vi "I2C_Core_[Top-Level].vi"() -> ()   [LabVIEW 2019]
doc: "I2C Core is a general FPGA VI for communicating with I2C devices.\n_____________________________________________________\nI2C Data transfers fit into three basic formats: \n\nThe first, a simple master-to-slave transfer, begins with the master generating a start condition. The master then sends the desired 7-bit slave address with the read/write bit cleared and begins the acknowledgment clock cycle. Once the ACK condition is observed, the cycle of writing data and reading ACK bits continues until the receiver either issues a NOACK or the transmitter completes the transfer and issues a STOP condition. \n\nThe second format, master-slave read, is similar to the previous format, except that the slave device immediately begins placing data onto the bus after the acknowledgment clock. \n\nThe last category is a combined format. Often this format is used when a device requires some initial configuration information in order to continue. Again, this format is similar to the previous two except that instead of issuing a stop condition, the transmitter issues a second start condition, followed by the slave address. You will often see this command used when accessing devices like serial EEPROMs. The first sequence is used to supply the device with the address that should be read, while the second start and clock sequence are used to clock the data back. \n\n\nTechnical Information Source:\nhttp://www.embedded.com/97/feat9711.htm\n_____________________________________________________\n\nWritten By: \nPeter Fuller\nplf Consulting, LLC\n258 Harvard St #324\nBrookline, MA 02446\n\nemail: peter@plfconsulting.com\nphone: 617.699.2201"
uses:
  Controls/i2c_state.ctl
  <vilib>/eio/EIONode/EIONode.xnode
  Instance           4 28Saved   I2C_Core_[Top-Level] .vi
  <vilib>/eio/EIOMethodNode/EIOMethodNode.xnode
  <vilib>/rvi/eio/common/nirviEmuTemplateMethod_errors.vi
panel:
  out "AI3":fxp<+/-,24,5>
  out "AI2":fxp<+/-,24,5>
  out "AI1":fxp<+/-,24,5>
  in  "Execute 2":bool
  in  "HalfCycle(Ticks) 2":u32=200
  in  "i2c_State 2":T1=enum."W_To_Device"
  in  "Address 2":u8 format="%08x"
  in  "10-bitAddress 2":u8 format="%08b"
  in  "TransmitDelay(Ticks) 2":u32=1000
  in  "Use_10-Bit_Address 2":bool
  in  "StartStopDelay(Ticks) 2":u32=1200
  in  "PostAddressDelay(Ticks) 2":u32=1200
  in  "NumBytesToWrite 2":i32
  in  "NumBytesToRead 2":i32
  out "error 2":errorcluster
  out "Status 2":i16
  in  "CMD/Param 2":u8 format="%.0x"
  out "Data 2":u8 format="%.0x"
  in  "MemoryAddress 2":u32
  in  "GetRead 2":bool
  in  "UpdateWrite 2":bool
  out "AI0":fxp<+/-,24,5>
  out "error":errorcluster
  in  "PostAddressDelay(Ticks)":u32=1200
  in  "StartStopDelay(Ticks)":u32=1200
  in  "NumBytesToRead":i32
  in  "NumBytesToWrite":i32
  in  "UpdateWrite":bool
  in  "GetRead":bool
  in  "CMD/Param":u8 format="%.0x"
  out "Data":u8 format="%.0x"
  in  "MemoryAddress":u32
  out "Status":i16
  in  "Use_10-Bit_Address":bool
  in  "TransmitDelay(Ticks)":u32=1000
  in  "10-bitAddress":u8 format="%08b"
  in  "Address":u8 format="%08x"
  in  "HalfCycle(Ticks)":u32=200
  in  "i2c_State":T1=enum."W_To_Device"
  in  "Execute":bool
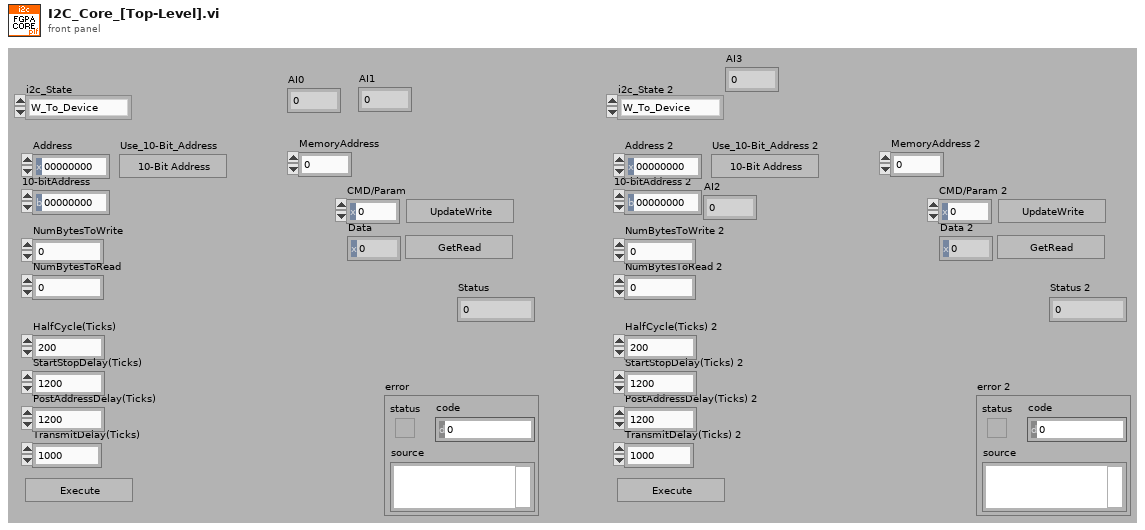
[diagram p1: front panel]
types:
  T1 = typedef "i2c_state.ctl" = enum16{"Monitor", "W_To_Device", "R_From_Device", "W/R_From_Device", "TerminateCore"}
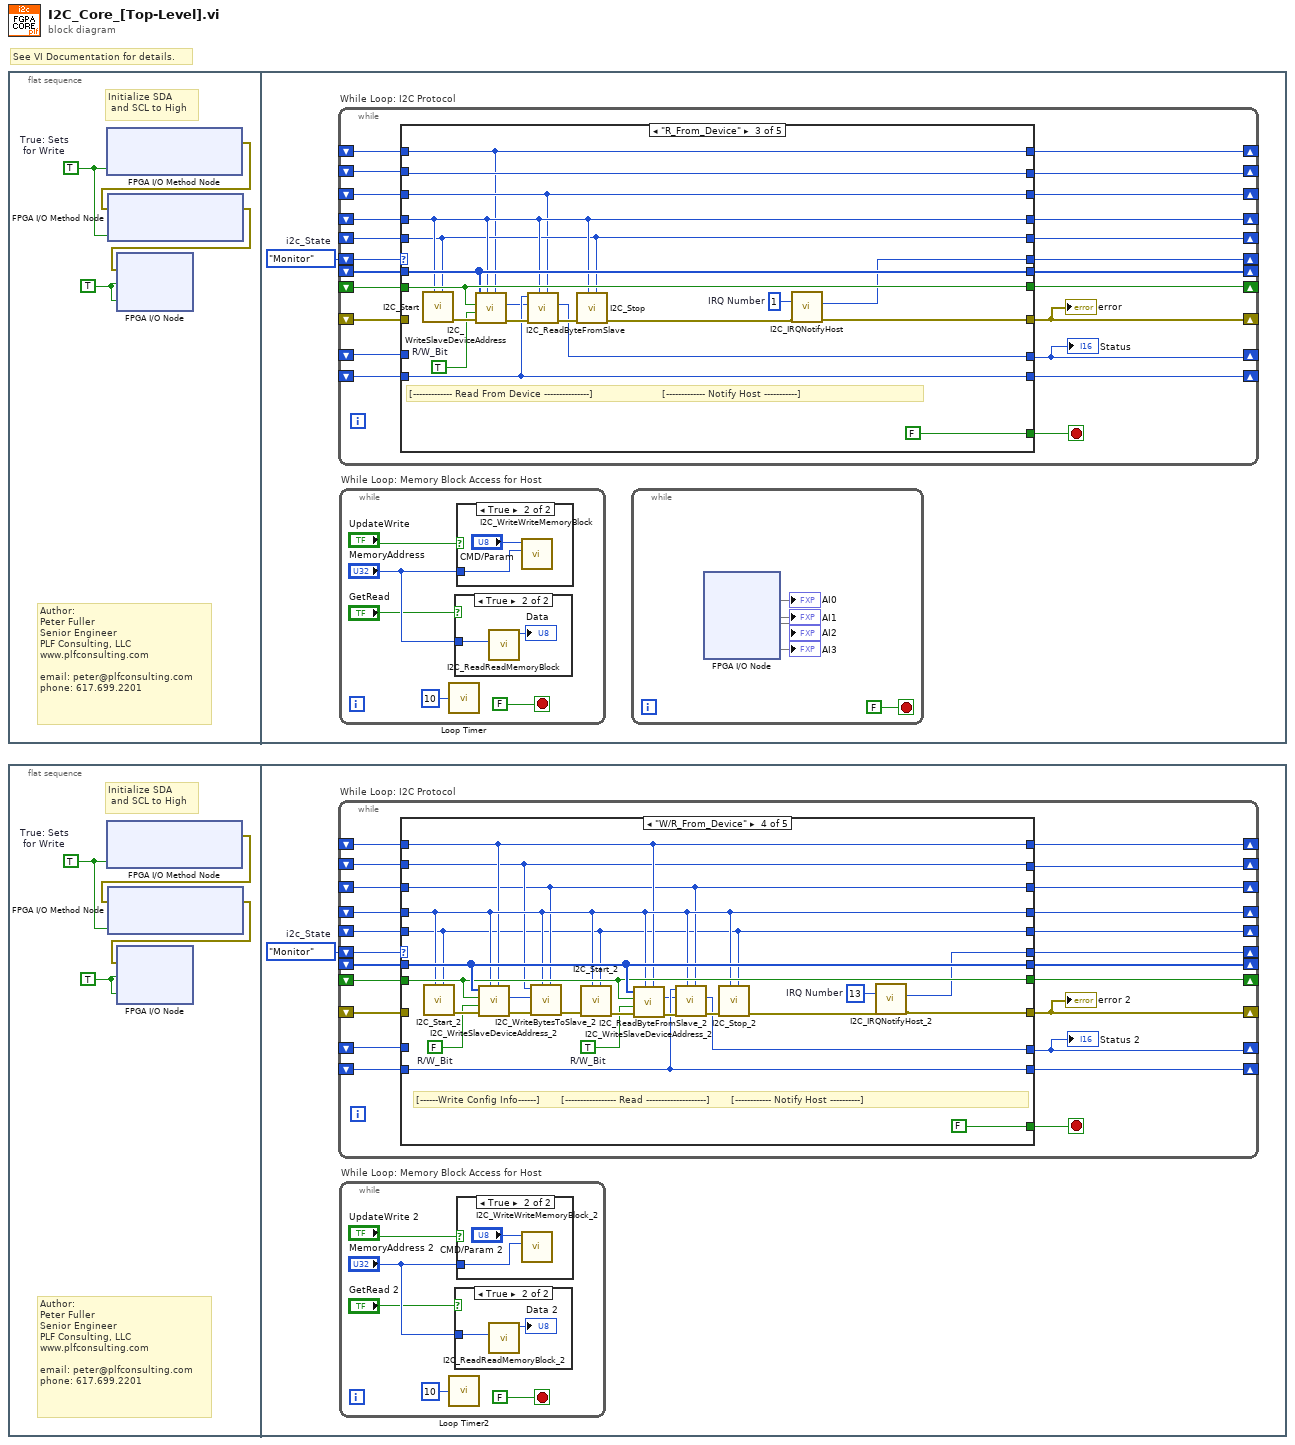
[diagram p0: block diagram]
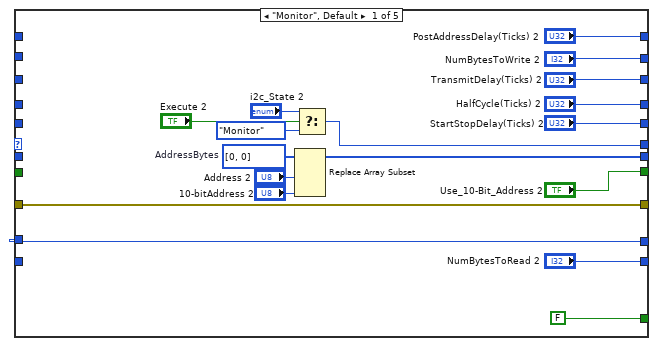
[diagram p4: hidden frame]
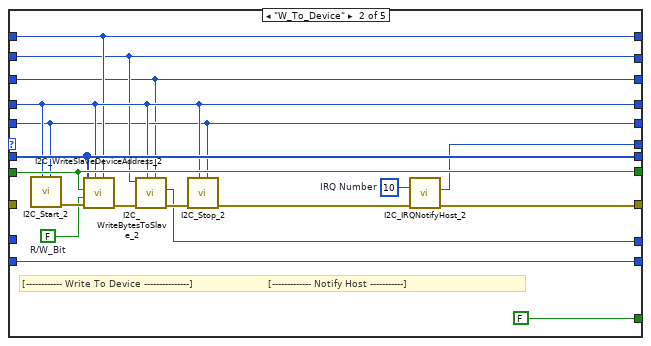
[diagram p5: hidden frame]
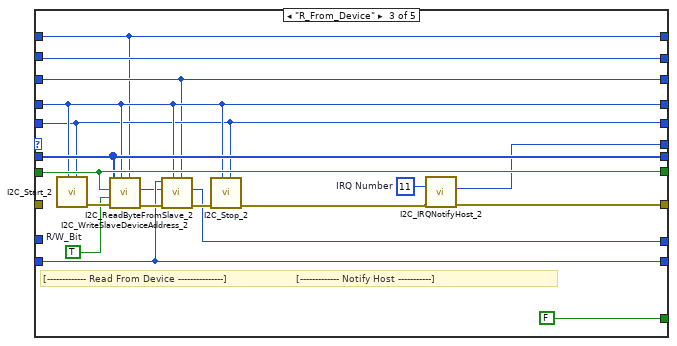
[diagram p6: hidden frame]
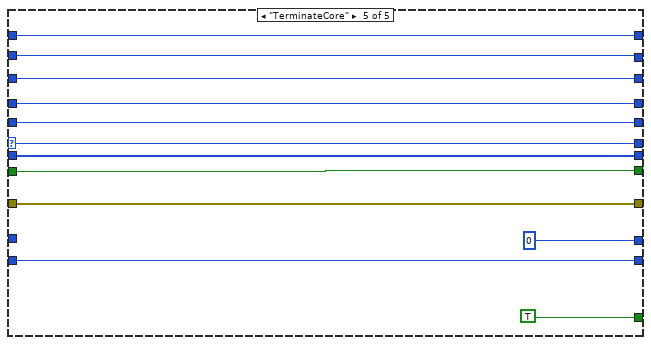
[diagram p7: hidden frame]
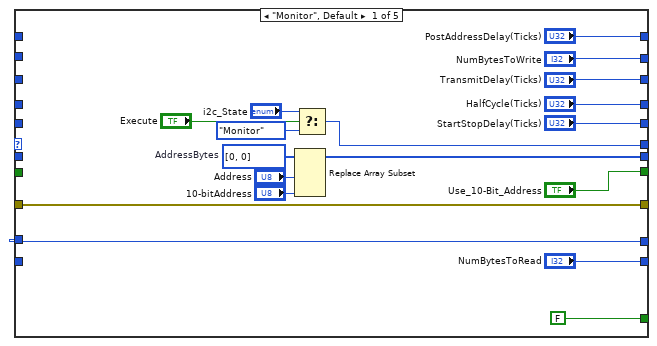
[diagram p10: hidden frame]
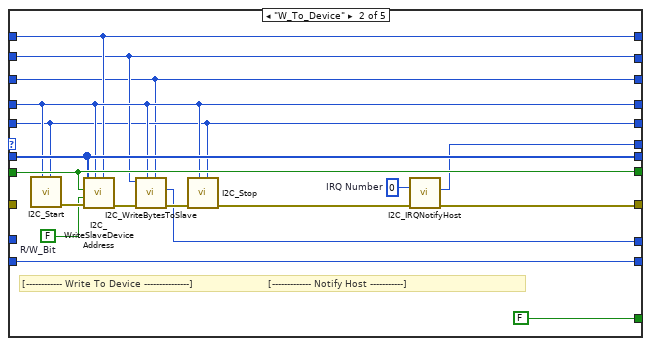
[diagram p11: hidden frame]
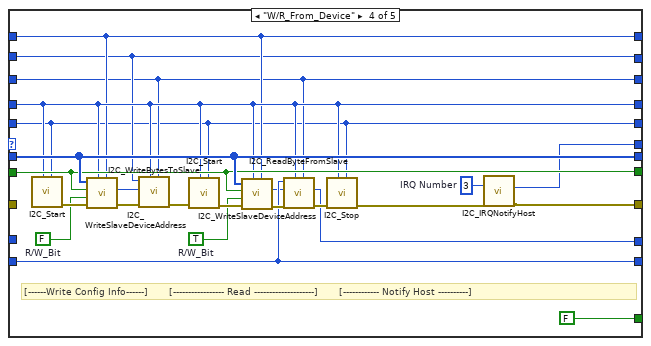
[diagram p12: hidden frame]
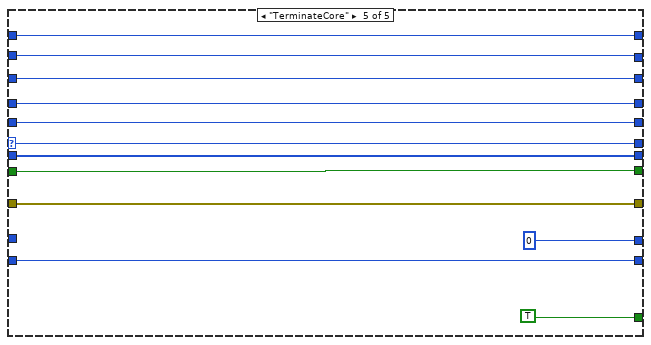
[diagram p13: hidden frame]
diagram:
  # "See VI Documentation for details."
  n1 = flat-sequence {
    frame #0 {
      w2 = TRUE  # True: Sets   for Write
      w4 = TRUE ("SDA")
      # "Author:\nPeter Fuller\nSenior Engineer\nPLF Consulting, LLC\nwww.plfconsulting.com\n\nemail: peter@plfconsulting.com\nphone: 617.699.2201"
      # "Initialize SDA\n and SCL to High"
      n2 = xnode "FPGA I/O Method Node"("Enable"=w2) -> ("error out"=w3:errorcluster)  [unwired: 2 in, 1 out]
      n3 = xnode "FPGA I/O Method Node"("error in"=w3, "Enable"=w2) -> ("error out"=w1:errorcluster)  [unwired: 1 in, 1 out]
      n4 = xnode "FPGA I/O Node"("error in"=w1, "SDA"=w4, "SCL"=w4) -> ()  [unwired: 2 in, 3 out]
    }
    frame #1 {
      w5 = i2c_state."Monitor"  # i2c_State
      n5 = while "While Loop: I2C Protocol" {
        shift-right: [w37] -> _
        shift-left: w5 -> [w38]
        shift-right: [w41] -> _
        shift-left: _ -> [w42]
        shift-right: [w22] -> _
        shift-left: _ -> [w40]
        shift-right: [w36] -> _
        shift-left: _ -> [w39]
        shift-right: [w35] -> _
        shift-left: _ -> [w34]
        shift-right: [w33] -> _
        shift-left: _ -> [w32]
        shift-right: [w30] -> _
        shift-left: _ -> [w26]
        shift-right: [w29] -> _
        shift-left: _ -> [w25]
        shift-right: [w28] -> _
        shift-left: _ -> [w23]
        shift-right: [w27] -> _
        shift-left: _ -> [w24]
        shift-right: [w21] -> _
        shift-left: _ -> [w20]
        stop <- w31 stop-if-true
        n6 = case shown="\"R_From_Device\"" w38 {
          selector: w38 -> [_ _ _ _ w126]
          tunnel: ["HalfCycle(Ticks)" w75 w92 w113 w128] -> w41
          tunnel: w42 -> [_ w75 w92 w113 w128]
          tunnel: [w56 w70 w79 w98 w126] -> w37
          tunnel: w40 -> [w44 _ _ _ w132]
          tunnel: [w44 w63 w80 w99 w132] -> w22
          tunnel: w39 -> [_ w76 w95 w118 w125]
          tunnel: [w52 w76 w95 w118 w125] -> w36
          tunnel: ["Use_10-Bit_Address" w77 w96 w117 w124] -> w35
          tunnel: w34 -> [_ w77 w96 w117 w124]
          tunnel: ["TransmitDelay(Ticks)" w64 w86 w106 w129] -> w33
          tunnel: w32 -> [_ w64 w86 w106 w129]
          tunnel: [FALSE FALSE FALSE FALSE TRUE] -> w31
          tunnel: w25 -> [_ w67 w89 w108 w130]
          tunnel: w24 -> [_ w66 w88 w107 w123]
          tunnel: w23 -> [_ w65 w87 w105 w127]
          tunnel: ["PostAddressDelay(Ticks)" w68 w85 w109 w131] -> w30
          tunnel: ["NumBytesToWrite" w67 w89 w108 w130] -> w29
          tunnel: ["StartStopDelay(Ticks)" w65 w87 w105 w127] -> w28
          tunnel: ["NumBytesToRead" w66 w88 w107 w123] -> w27
          tunnel: w26 -> [_ w68 w85 w109 w131]
          tunnel: [w43 w62 w84 w104 i16 0 ("Status")] -> w21
          tunnel: w20 -> [w43 _ _ _ _]
          frame "Monitor", Default {
            w55 = u8[] [0, 0]  # AddressBytes
            n7 = Replace Array Subset(array=w55, new element #1="Address", new element #2="10-bitAddress") -> (w52:u8[])  [unwired: 2 in]
            n8 = Select(t="i2c_State", s="Execute", f=i2c_state."Monitor") -> (s? t:f=w56:T1)
          }
          frame "W_To_Device" {
            w61 = u8 0  # IRQ Number
            w71 = FALSE  # R/W_Bit
            # "[------------ Write To Device ---------------]                         [------------- Notify Host -----------]"
            n9 = call "I2C_Start.vi"("TransmitDelay(Ticks)"=w65, "HalfCycle(Ticks)"=w75) -> ("error out"=w74:errorcluster)  [unwired: 2 in, 7 out]
            n10 = call "I2C_WriteSlaveDeviceAddress.vi"("PostAddressDelay(Ticks)"=w68, "HalfCycle(Ticks)"=w75, "error in"=w74, "R/W_Bit"=w71, "10-Bit Address"=w77, "AddressBits"=w76) -> ("error out"=w78:errorcluster)  [unwired: 5 out]
            n11 = call "I2C_WriteBytesToSlave.vi"("InterByteTransmitDelay(Ticks)"=w64, "HalfCycle(Ticks)"=w75, "error in"=w78, "NumBytesToWrite"=w67) -> ("error out"=w73:errorcluster, "Status"=w62:i16)  [unwired: 1 in, 5 out]
            n12 = call "I2C_Stop.vi"("TransmitDelay(Ticks)"=w65, "HalfCycle(Ticks)"=w75, "error in"=w73) -> ("error out"=w69:errorcluster)  [unwired: 1 in, 7 out]
            n13 = call "I2C_IRQNotifyHost.vi"("error out in"=w69, "IRQ Number"=w61) -> ("error out"=w63:errorcluster, "i2c_State"=w70:T1)  [unwired: 8 out]
          }
          frame "R_From_Device" {
            w82 = u8 1  # IRQ Number
            w90 = TRUE  # R/W_Bit
            # "[------------- Read From Device ---------------]                       [------------- Notify Host -----------]"
            n14 = call "I2C_Start.vi"("TransmitDelay(Ticks)"=w87, "HalfCycle(Ticks)"=w92) -> ("error out"=w94:errorcluster)  [unwired: 2 in, 7 out]
            n15 = call "I2C_WriteSlaveDeviceAddress.vi"("PostAddressDelay(Ticks)"=w85, "HalfCycle(Ticks)"=w92, "error in"=w94, "R/W_Bit"=w90, "10-Bit Address"=w96, "AddressBits"=w95) -> ("error out"=w97:errorcluster, "Status"=w83:i16)  [unwired: 4 out]
            n16 = call "I2C_ReadByteFromSlave.vi"("InterByteTransmitDelay(Ticks)"=w86, "HalfCycle(Ticks)"=w92, "error in"=w97, "StatusIn"=w83, "NumBytesToRead"=w88) -> ("error out"=w93:errorcluster, "Status"=w84:i16)  [unwired: 5 out]
            n17 = call "I2C_Stop.vi"("TransmitDelay(Ticks)"=w87, "HalfCycle(Ticks)"=w92, "error in"=w93) -> ("error out"=w81:errorcluster)  [unwired: 1 in, 7 out]
            n18 = call "I2C_IRQNotifyHost.vi"("error out in"=w81, "IRQ Number"=w82) -> ("error out"=w80:errorcluster, "i2c_State"=w79:T1)  [unwired: 8 out]
          }
          frame "W/R_From_Device" {
            w101 = u8 3  # IRQ Number
            w110 = TRUE  # R/W_Bit
            w111 = FALSE  # R/W_Bit
            # "[------Write Config Info------]       [----------------- Read --------------------]       [------------ Notify Host ----------]"
            n19 = call "I2C_Start.vi"("TransmitDelay(Ticks)"=w105, "HalfCycle(Ticks)"=w113) -> ("error out"=w121:errorcluster)  [unwired: 2 in, 7 out]
            n20 = call "I2C_WriteSlaveDeviceAddress.vi"("PostAddressDelay(Ticks)"=w109, "HalfCycle(Ticks)"=w113, "error in"=w121, "R/W_Bit"=w111, "10-Bit Address"=w117, "AddressBits"=w118) -> ("error out"=w114:errorcluster, "Status"=w103:i16)  [unwired: 4 out]
            n21 = call "I2C_WriteBytesToSlave.vi"("InterByteTransmitDelay(Ticks)"=w106, "HalfCycle(Ticks)"=w113, "error in"=w114, "StatusIn"=w103, "NumBytesToWrite"=w108) -> ("error out"=w115:errorcluster)  [unwired: 6 out]
            n22 = call "I2C_Start.vi"("TransmitDelay(Ticks)"=w105, "HalfCycle(Ticks)"=w113, "error in"=w115) -> ("error out"=w119:errorcluster)  [unwired: 1 in, 7 out]
            n23 = call "I2C_WriteSlaveDeviceAddress.vi"("PostAddressDelay(Ticks)"=w109, "HalfCycle(Ticks)"=w113, "error in"=w119, "R/W_Bit"=w110, "10-Bit Address"=w117, "AddressBits"=w118) -> ("error out"=w116:errorcluster, "Status"=w102:i16)  [unwired: 4 out]
            n24 = call "I2C_ReadByteFromSlave.vi"("InterByteTransmitDelay(Ticks)"=w106, "HalfCycle(Ticks)"=w113, "error in"=w116, "StatusIn"=w102, "NumBytesToRead"=w107) -> ("error out"=w120:errorcluster, "Status"=w104:i16)  [unwired: 5 out]
            n25 = call "I2C_Stop.vi"("TransmitDelay(Ticks)"=w105, "HalfCycle(Ticks)"=w113, "error in"=w120) -> ("error out"=w100:errorcluster)  [unwired: 1 in, 7 out]
            n26 = call "I2C_IRQNotifyHost.vi"("error out in"=w100, "IRQ Number"=w101) -> ("error out"=w99:errorcluster, "i2c_State"=w98:T1)  [unwired: 8 out]
          }
          frame "TerminateCore" {
          }
        }
        "error" <- w22
        "Status" <- w21
      }
      n27 = while "While Loop: Memory Block Access for Host" {
        stop <- FALSE stop-if-true
        n28 = call "Loop Timer"("Count(Ticks)"=u16 10) -> ()  [unwired: 1 out]
        n29 = case shown="True" "GetRead" {
          tunnel: "MemoryAddress" -> [_ w17]
          frame False {
          }
          frame True {
            n30 = call "I2C_ReadReadMemoryBlock.vi"("MemoryAddress"=w17) -> ("Data"=→"Data":u8)  [unwired: 1 in, 9 out]
          }
        }
        n31 = case shown="True" "UpdateWrite" {
          tunnel: "MemoryAddress" -> [_ w19]
          frame False {
          }
          frame True {
            n32 = call "I2C_WriteWriteMemoryBlock.vi"("MemoryAddress"=w19, "Data"="CMD/Param") -> ()  [unwired: 1 in, 9 out]
          }
        }
      }
      n33 = while {
        stop <- FALSE stop-if-true
        n34 = xnode "FPGA I/O Node"() -> ("AI0"=→"AI0", "AI1"=→"AI1", "AI2"=→"AI2", "AI3"=→"AI3")  [unwired: 4 in, 4 out]
      }
    }
  }
  n35 = flat-sequence {
    frame #0 {
      w135 = TRUE  # True: Sets   for Write
      w137 = TRUE ("SDA")
      # "Author:\nPeter Fuller\nSenior Engineer\nPLF Consulting, LLC\nwww.plfconsulting.com\n\nemail: peter@plfconsulting.com\nphone: 617.699.2201"
      # "Initialize SDA\n and SCL to High"
      n36 = xnode "FPGA I/O Method Node"("Enable"=w135) -> ("error out"=w136:errorcluster)  [unwired: 2 in, 1 out]
      n37 = xnode "FPGA I/O Method Node"("error in"=w136, "Enable"=w135) -> ("error out"=w134:errorcluster)  [unwired: 1 in, 1 out]
      n38 = xnode "FPGA I/O Node"("error in"=w134, "SDA2"=w137, "SCL2"=w137) -> ()  [unwired: 2 in, 3 out]
    }
    frame #1 {
      w138 = i2c_state."Monitor"  # i2c_State
      n39 = while "While Loop: I2C Protocol" {
        shift-right: [w165] -> _
        shift-left: w138 -> [w166]
        shift-right: [w169] -> _
        shift-left: _ -> [w170]
        shift-right: [w150] -> _
        shift-left: _ -> [w168]
        shift-right: [w164] -> _
        shift-left: _ -> [w167]
        shift-right: [w163] -> _
        shift-left: _ -> [w162]
        shift-right: [w161] -> _
        shift-left: _ -> [w160]
        shift-right: [w158] -> _
        shift-left: _ -> [w154]
        shift-right: [w157] -> _
        shift-left: _ -> [w153]
        shift-right: [w156] -> _
        shift-left: _ -> [w151]
        shift-right: [w155] -> _
        shift-left: _ -> [w152]
        shift-right: [w149] -> _
        shift-left: _ -> [w148]
        stop <- w159 stop-if-true
        n40 = case shown="\"W/R_From_Device\"" w166 {
          selector: w166 -> [_ _ _ _ w254]
          tunnel: ["HalfCycle(Ticks) 2" w203 w220 w241 w256] -> w169
          tunnel: w170 -> [_ w203 w220 w241 w256]
          tunnel: [w184 w198 w207 w226 w254] -> w165
          tunnel: w168 -> [w172 _ _ _ w260]
          tunnel: [w172 w191 w208 w227 w260] -> w150
          tunnel: w167 -> [_ w204 w223 w246 w253]
          tunnel: [w180 w204 w223 w246 w253] -> w164
          tunnel: ["Use_10-Bit_Address 2" w205 w224 w245 w252] -> w163
          tunnel: w162 -> [_ w205 w224 w245 w252]
          tunnel: ["TransmitDelay(Ticks) 2" w192 w214 w234 w257] -> w161
          tunnel: w160 -> [_ w192 w214 w234 w257]
          tunnel: [FALSE FALSE FALSE FALSE TRUE] -> w159
          tunnel: w153 -> [_ w195 w217 w236 w258]
          tunnel: w152 -> [_ w194 w216 w235 w251]
          tunnel: w151 -> [_ w193 w215 w233 w255]
          tunnel: ["PostAddressDelay(Ticks) 2" w196 w213 w237 w259] -> w158
          tunnel: ["NumBytesToWrite 2" w195 w217 w236 w258] -> w157
          tunnel: ["StartStopDelay(Ticks) 2" w193 w215 w233 w255] -> w156
          tunnel: ["NumBytesToRead 2" w194 w216 w235 w251] -> w155
          tunnel: w154 -> [_ w196 w213 w237 w259]
          tunnel: [w171 w190 w212 w232 i16 0 ("Status")] -> w149
          tunnel: w148 -> [w171 _ _ _ _]
          frame "Monitor", Default {
            w183 = u8[] [0, 0]  # AddressBytes
            n41 = Replace Array Subset(array=w183, new element #1="Address 2", new element #2="10-bitAddress 2") -> (w180:u8[])  [unwired: 2 in]
            n42 = Select(t="i2c_State 2", s="Execute 2", f=i2c_state."Monitor") -> (s? t:f=w184:T1)
          }
          frame "W_To_Device" {
            w189 = u8 10  # IRQ Number
            w199 = FALSE  # R/W_Bit
            # "[------------ Write To Device ---------------]                         [------------- Notify Host -----------]"
            n43 = call "I2C_Start_2.vi"("TransmitDelay(Ticks)"=w193, "HalfCycle(Ticks)"=w203) -> ("error out"=w202:errorcluster)  [unwired: 9 in]
            n44 = call "I2C_WriteSlaveDeviceAddress_2.vi"("PostAddressDelay(Ticks)"=w196, "HalfCycle(Ticks)"=w203, "error in"=w202, "R/W_Bit"=w199, "10-Bit Address"=w205, "AddressBits"=w204) -> ("error out"=w206:errorcluster)  [unwired: 4 in, 1 out]
            n45 = call "I2C_WriteBytesToSlave_2.vi"("InterByteTransmitDelay(Ticks)"=w192, "HalfCycle(Ticks)"=w203, "error in"=w206, "NumBytesToWrite"=w195) -> ("error out"=w201:errorcluster, "Status"=w190:i16)  [unwired: 6 in]
            n46 = call "I2C_Stop_2.vi"("TransmitDelay(Ticks)"=w193, "HalfCycle(Ticks)"=w203, "error in"=w201) -> ("error out"=w197:errorcluster)  [unwired: 8 in]
            n47 = call "I2C_IRQNotifyHost_2.vi"("error out in"=w197, "IRQ Number"=w189) -> ("error out"=w191:errorcluster, "i2c_State"=w198:T1)  [unwired: 8 in]
          }
          frame "R_From_Device" {
            w210 = u8 11  # IRQ Number
            w218 = TRUE  # R/W_Bit
            # "[------------- Read From Device ---------------]                       [------------- Notify Host -----------]"
            n48 = call "I2C_Start_2.vi"("TransmitDelay(Ticks)"=w215, "HalfCycle(Ticks)"=w220) -> ("error out"=w222:errorcluster)  [unwired: 9 in]
            n49 = call "I2C_WriteSlaveDeviceAddress_2.vi"("PostAddressDelay(Ticks)"=w213, "HalfCycle(Ticks)"=w220, "error in"=w222, "R/W_Bit"=w218, "10-Bit Address"=w224, "AddressBits"=w223) -> ("error out"=w225:errorcluster, "Status"=w211:i16)  [unwired: 4 in]
            n50 = call "I2C_ReadByteFromSlave_2.vi"("InterByteTransmitDelay(Ticks)"=w214, "HalfCycle(Ticks)"=w220, "error in"=w225, "StatusIn"=w211, "NumBytesToRead"=w216) -> ("error out"=w221:errorcluster, "Status"=w212:i16)  [unwired: 5 in]
            n51 = call "I2C_Stop_2.vi"("TransmitDelay(Ticks)"=w215, "HalfCycle(Ticks)"=w220, "error in"=w221) -> ("error out"=w209:errorcluster)  [unwired: 8 in]
            n52 = call "I2C_IRQNotifyHost_2.vi"("error out in"=w209, "IRQ Number"=w210) -> ("error out"=w208:errorcluster, "i2c_State"=w207:T1)  [unwired: 8 in]
          }
          frame "W/R_From_Device" {
            w229 = u8 13  # IRQ Number
            w238 = TRUE  # R/W_Bit
            w239 = FALSE  # R/W_Bit
            # "[------Write Config Info------]       [----------------- Read --------------------]       [------------ Notify Host ----------]"
            n53 = call "I2C_Start_2.vi"("TransmitDelay(Ticks)"=w233, "HalfCycle(Ticks)"=w241) -> ("error out"=w249:errorcluster)  [unwired: 9 in]
            n54 = call "I2C_WriteSlaveDeviceAddress_2.vi"("PostAddressDelay(Ticks)"=w237, "HalfCycle(Ticks)"=w241, "error in"=w249, "R/W_Bit"=w239, "10-Bit Address"=w245, "AddressBits"=w246) -> ("error out"=w242:errorcluster, "Status"=w231:i16)  [unwired: 4 in]
            n55 = call "I2C_WriteBytesToSlave_2.vi"("InterByteTransmitDelay(Ticks)"=w234, "HalfCycle(Ticks)"=w241, "error in"=w242, "StatusIn"=w231, "NumBytesToWrite"=w236) -> ("error out"=w243:errorcluster)  [unwired: 5 in, 1 out]
            n56 = call "I2C_Start_2.vi"("TransmitDelay(Ticks)"=w233, "HalfCycle(Ticks)"=w241, "error in"=w243) -> ("error out"=w247:errorcluster)  [unwired: 8 in]
            n57 = call "I2C_WriteSlaveDeviceAddress_2.vi"("PostAddressDelay(Ticks)"=w237, "HalfCycle(Ticks)"=w241, "error in"=w247, "R/W_Bit"=w238, "10-Bit Address"=w245, "AddressBits"=w246) -> ("error out"=w244:errorcluster, "Status"=w230:i16)  [unwired: 4 in]
            n58 = call "I2C_ReadByteFromSlave_2.vi"("InterByteTransmitDelay(Ticks)"=w234, "HalfCycle(Ticks)"=w241, "error in"=w244, "StatusIn"=w230, "NumBytesToRead"=w235) -> ("error out"=w248:errorcluster, "Status"=w232:i16)  [unwired: 5 in]
            n59 = call "I2C_Stop_2.vi"("TransmitDelay(Ticks)"=w233, "HalfCycle(Ticks)"=w241, "error in"=w248) -> ("error out"=w228:errorcluster)  [unwired: 8 in]
            n60 = call "I2C_IRQNotifyHost_2.vi"("error out in"=w228, "IRQ Number"=w229) -> ("error out"=w227:errorcluster, "i2c_State"=w226:T1)  [unwired: 8 in]
          }
          frame "TerminateCore" {
          }
        }
        "error 2" <- w150
        "Status 2" <- w149
      }
      n61 = while "While Loop: Memory Block Access for Host" {
        stop <- FALSE stop-if-true
        n62 = call "Loop Timer2"("Count(Ticks)"=u16 10) -> ()  [unwired: 1 out]
        n63 = case shown="True" "GetRead 2" {
          tunnel: "MemoryAddress 2" -> [_ w145]
          frame False {
          }
          frame True {
            n64 = call "I2C_ReadReadMemoryBlock_2.vi"("MemoryAddress"=w145) -> ("Data"=→"Data 2":u8)  [unwired: 9 in, 1 out]
          }
        }
        n65 = case shown="True" "UpdateWrite 2" {
          tunnel: "MemoryAddress 2" -> [_ w147]
          frame False {
          }
          frame True {
            n66 = call "I2C_WriteWriteMemoryBlock_2.vi"("MemoryAddress"=w147, "Data"="CMD/Param 2") -> ()  [unwired: 9 in, 1 out]
          }
        }
      }
    }
  }
